vi "SRU2P（U8）.vi"(5 "初始值":u8, 6 "复位":bool, 7 "启用（T）":bool=TRUE, 9 "Yi":u8, 10 "Xi":u8) -> (1 "Yi-1":u8, 2 "Xi-1":u8)   [LabVIEW 2012]
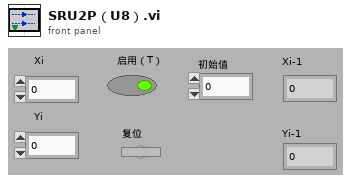
[diagram p1: front panel]
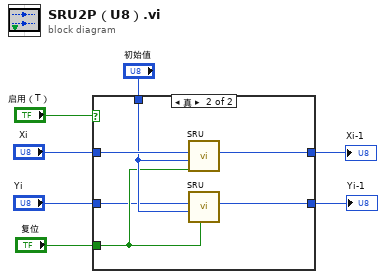
[diagram p0: block diagram]
diagram:
  n1 = case shown="真" "启用（T）" {
    tunnel: "复位" -> [_ w13]
    tunnel: "Xi" -> [w9 w15]
    tunnel: [w9 w12] -> w5
    tunnel: "初始值" -> [_ w14]
    tunnel: [w8 w11] -> w2
    tunnel: "Yi" -> [w8 w10]
    frame False {
    }
    frame True {
      n2 = call-poly "SRU.vi"("复位"=w13, "初始值"=w14, "输入"=w15) -> ("上次值"=w12:u8)  [unwired: 6 in, 2 out]
      n3 = call-poly "SRU.vi"("复位"=w13, "初始值"=w14, "输入"=w10) -> ("上次值"=w11:u8)  [unwired: 6 in, 2 out]
    }
  }
  "Xi-1" <- w5
  "Yi-1" <- w2
